vi "query_temperature(SubVI).vi"(8 "error in (no error)":errorcluster, 11 "VISA Refnum in":refnum<visa-resource-name>) -> (0 "error out":errorcluster, 2 "read buffer":string, 3 "VISA resource name out":refnum<visa-resource-name>)   [LabVIEW 2018]
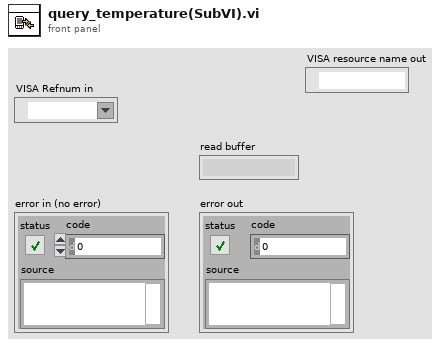
[diagram p1: front panel]
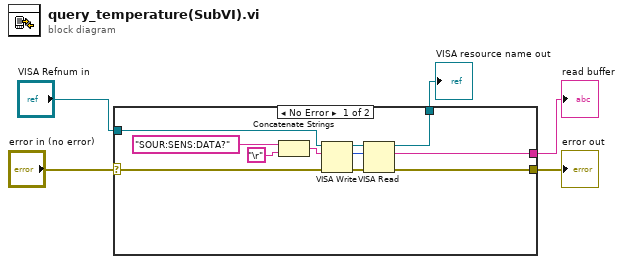
[diagram p0: block diagram]
diagram:
  n1 = case shown="No Error" "error in (no error)" {
    selector: "error in (no error)" -> [w7 w18]
    tunnel: [w15 _] -> w5
    tunnel: [w14 w18] -> w4
    tunnel: "VISA Refnum in" -> [w8 w17]
    tunnel: [w6 w17] -> w1
    frame No Error {
      n2 = Concatenate Strings("SOUR:SENS:DATA?" ("string"), "\r") -> (w11:string)
      n3 = VISA Write(VISA resource name=w8, write buffer=w11, error in (no error)=w7) -> (VISA resource name out=w12:refnum<visa-resource-name>, return count=w16:u32, error out=w13:errorcluster)
      n4 = VISA Read(VISA resource name=w12, byte count=w16, error in (no error)=w13) -> (VISA resource name out=w6:refnum<visa-resource-name>, read buffer=w15:string, error out=w14:errorcluster)  [unwired: 1 out]
    }
    frame Error {
    }
  }
  "read buffer" <- w5
  "error out" <- w4
  "VISA resource name out" <- w1
